vi "Map to Solution Grid.vi"(8 "error in (no error)":errorcluster, 11 "Grassfire Algorithm in":refnum<class "Grassfire Algorithm.lvclass">) -> (0 "error out":errorcluster, 3 "Grassfire Algorithm out":refnum<class "Grassfire Algorithm.lvclass">)   [LabVIEW 2019, in "Grassfire Algorithm.lvclass"]
uses:
  Grassfire Algorithm.lvclass
  Solution Grid Cell--cluster.ctl
  Solution--picture ring.ctl
  Grassfire Algorithm.lvclass/Grassfire Algorithm.ctl
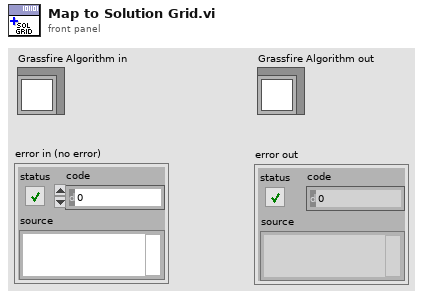
[diagram p1: front panel]
types:
  T1 = typedef "Grassfire Algorithm.lvclass/Solution Grid Cell--cluster.ctl" = cluster{"Picture":T2, "Value":string}
  T2 = typedef "Grassfire Algorithm.lvclass/Solution--picture ring.ctl" = i64
  T3 = typedef "Grassfire Algorithm.lvclass/Index Column Row--cluster.ctl" = cluster{"Row":i32, "Column":i32}
  T4 = typedef "Grassfire Algorithm.lvclass/Solution Grid Cell Private--cluster.ctl" = cluster{"Picture":T2, "Value":dbl}
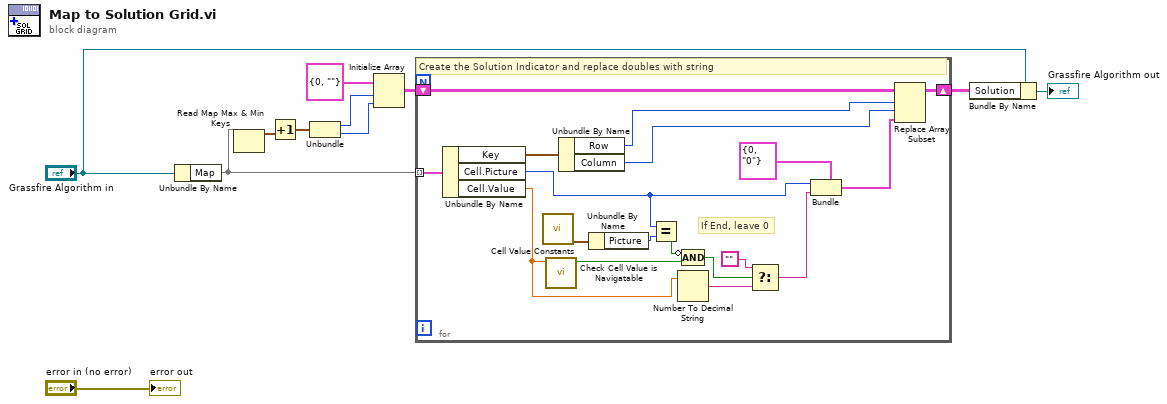
[diagram p0: block diagram]
diagram:
  n1 = Unbundle By Name("Grassfire Algorithm in") -> ("Map"=w4:map{T3, T4})
  n2 = Read Map Max & Min Keys(11:w4) -> (3:w7:T3)  [unwired: 1 out]
  n3 = Increment(x=w7) -> (x+1=w8:T3)
  n4 = Unbundle(w8) -> ("Row"=w9:i32, "Column"=w10:i32)
  n5 = Initialize Array(T1 {"Picture"=0, "Value"=""} ("Cell"), w9, w10) -> (w11:T1[][])
  n6 = for {
    tunnel: w4 -> [w29] mode=indexing
    shift-right: [w26] -> w1
    shift-left: w11 -> [w27]
    # "If End, leave 0"
    # "Create the Solution Indicator and replace doubles with string"
    n7 = Unbundle By Name(w29) -> ("Key"=w28:T3, "Cell.Picture"=w14:T2, "Cell.Value"=w17:dbl)
    n8 = call "Cell Value Constants.vi"() -> ("End"=w16:T4)  [unwired: 8 in, 3 out]
    n9 = call "Check Cell Value is Navigatable.vi"("Value"=w17) -> ("Invalid Cell?"=w18:bool)  [unwired: 10 in]
    n10 = Unbundle By Name(w28) -> ("Row"=w25:i32, "Column"=w24:i32)
    n11 = Unbundle By Name(w16) -> ("Picture"=w15:T2)
    n12 = Equal?(x=w14, y=w15) -> (x = y?=w12:bool)
    n13 = Number To Decimal String(number=w17) -> (decimal integer string=w20:string)  [unwired: 1 in]
    n14 = Compound Arithmetic op=AND(invert w12, w18) -> (w13:bool)
    n15 = Select(t="", s=w13, f=w20) -> (s? t:f=w19:string)
    n16 = Bundle(cluster=T1 {"Picture"=0, "Value"="0"} ("new element/subarray"), "Picture"=w14, "Value"=w19) -> (w22:T1)
    n17 = Replace Array Subset(array=w27, new element=w22, index (row)=w25, index (col)=w24) -> (w26:T1[][])
  }
  n18 = Bundle By Name(cluster="Grassfire Algorithm in", "Solution"=w1) -> (→"Grassfire Algorithm out":refnum<class "Grassfire Algorithm.lvclass">)
  "error out" <- "error in (no error)"
